vi "PH_Trendviewer_Powermeter.ProcCases.vi"(0 "i ref in":refnum<vi>, 1 "selector":string, 2 "Data":T1, 3 "call cluster":T2={"Object"="", "Selector"="", "CallType"=enum."synchronous", "Async Object"="", "Async Selector"="", "Data Descriptor"="", "Data"=[], "Error #"=0, "Expire"=0}, 5 "error in (no error)":errorcluster) -> (14 "i ref out":refnum<vi>, 17 "answer cluster":T2={"Object"="", "Selector"="", "CallType"=enum."synchronous", "Async Object"="", "Async Selector"="", "Data Descriptor"="", "Data"=[], "Error #"=0, "Expire"=0}, 19 "error out":errorcluster)   [LabVIEW 2014, in "PH_Trendviewer_Powermeter.lvlib"]
doc: "This method is called by a process from within the default case in the event loop. The methods of a class that are linked to events will be called from THIS method. Add your code here."
uses:
  PH_Trendviewer_Powermeter.lvlib
  CS_Core/CSSystem/CoreDefs/CoreDefs.call_type.ctl
  CS_Core/BaseProcess/BaseProcess.descriptor string definition.ctl
  CS_Core/CSSystem/CoreDefs/CoreDefs.rawDataType.ctl
  CS_Core/CSSystem/CoreLib/CoreLib.byte array 2 short.vi
  CS_Core/CSSystem/CoreLib/CoreLib.string 2 byte array.vi
  CS_Core/CSSystem/CoreLib/CoreLib.lvlib
  CS_Core/BaseProcess/BaseProcess.lvlib
  PH_Basics/PH_PSDBWriter/PH_PSDBWriter.lvlib
  CS_Core/CAEObj/CAEObj.lvlib
  PH_Basics/PH_Common/PH_Common.lvlib
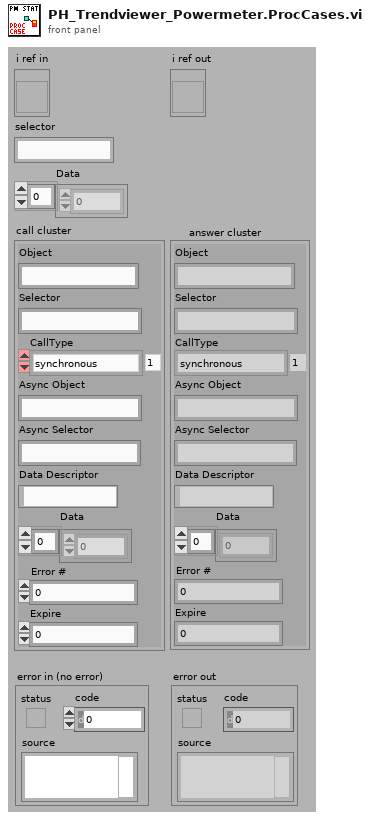
[diagram p1: front panel]
types:
  T1 = typedef "CoreDefs.rawDataType.ctl" = i8[]
  T2 = typedef "CoreDefs.call_type.ctl" = cluster{"Object":string, "Selector":string, "CallType":enum16{"simple", "synchronous", "asynchronous"}, "Async Object":string, "Async Selector":string, "Data Descriptor":T3, "Data":T1, "Error #":i32, "Expire":u32}
  T3 = typedef "BaseProcess.lvlib/BaseProcess.descriptor string definition.ctl" = string
  T4 = typedef "PH_Trendviewer_Powermeter.lvlib/PH_Trendviewer_Powermeter.i attribute.ctl" = cluster{"GUI Refs ":cluster{"Status":refnum<vi>, "Result Graph":refnum<vi>, "Mean Data":refnum<vi>, "Std Dev Data":refnum<vi>, "Dummy Mean":refnum<vi>, "Dummy Std Dev":refnum<vi>, "Export Data":refnum<vi>, "Stat or Trend":refnum<vi>, "Delete":refnum<vi>, "Powermeter":refnum<vi>, "Start":refnum<vi>}, "Powermeter":string, "Stat or Trend":bool, "Start":bool, "Data":cluster{"Time Stamp":timestamp, "Energy [J]":dbl}[], "Datasets strored":i32, "Dataarray Size":i32}
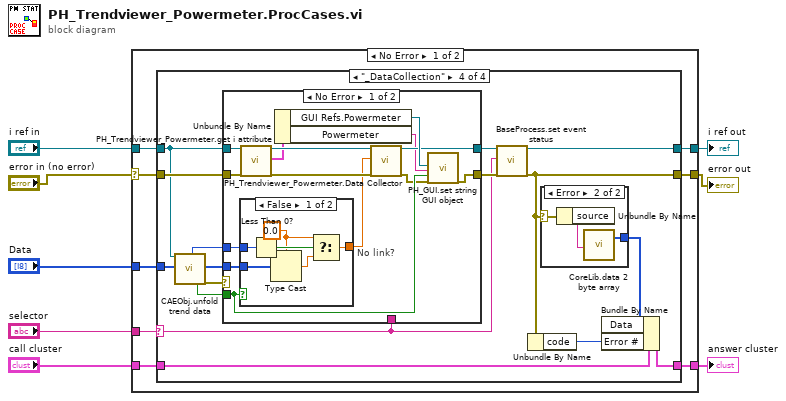
[diagram p0: block diagram]
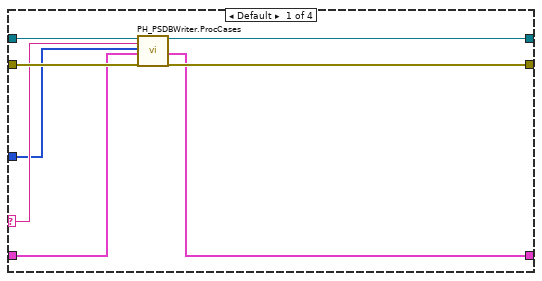
[diagram p2: hidden frame]
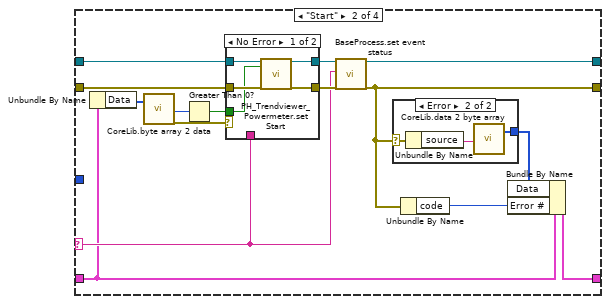
[diagram p3: hidden frame]
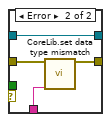
[diagram p5: hidden frame]
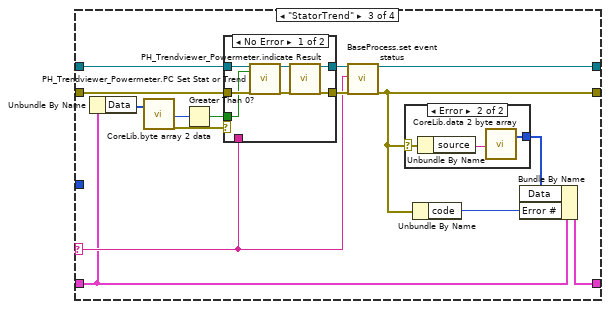
[diagram p6: hidden frame]
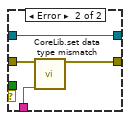
[diagram p8: hidden frame]
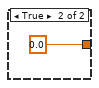
[diagram p10: hidden frame]
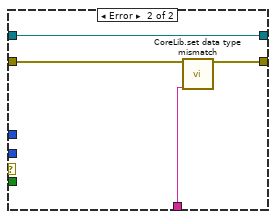
[diagram p11: hidden frame]
diagram:
  n1 = case shown="No Error" "error in (no error)" {
    selector: "error in (no error)" -> [w9 w126]
    tunnel: "selector" -> [w16 _]
    tunnel: [w15 w125] -> w7
    tunnel: "call cluster" -> [w14 w125]
    tunnel: "i ref in" -> [w13 w127]
    tunnel: [w12 w127] -> w5
    tunnel: [w11 w126] -> w4
    tunnel: "Data" -> [w10 _]
    frame No Error {
      n2 = case shown="\"_DataCollection\"" w16 {
        selector: w16 -> [w19 w28 w55 w89]
        tunnel: w13 -> [w18 w32 w59 w85]
        tunnel: [w24 w30 w57 w91] -> w12
        tunnel: w14 -> [w20 w27 w54 w88]
        tunnel: [w21 w26 w53 w87] -> w15
        tunnel: w9 -> [w23 w31 w58 w92]
        tunnel: [w22 w29 w56 w90] -> w11
        tunnel: w10 -> [w17 _ _ w86]
        frame Default {
          n3 = call "PH_PSDBWriter.ProcCases.vi"("i ref in"=w18, "selector"=w19, "Data"=w17, "call cluster"=w20, "error in"=w23) -> ("i ref out"=w24:refnum<vi>, "answer cluster"=w21:T2, "error out"=w22:errorcluster)  [unwired: 12 in]
        }
        frame "Start" {
          n4 = Unbundle By Name(w27) -> ("Data"=w35:T1)
          n5 = call-poly "CoreLib.byte array 2 data.vi"("byteArray"=w35) -> ("i16"=w36:i16, "error out"=w25:errorcluster)  [unwired: 16 in, 1 out]
          n6 = Greater Than 0?(x=w36) -> (x > 0?=w37:bool)
          n7 = case shown="No Error" w25 {
            tunnel: [w47 w51] -> w33
            tunnel: w32 -> [w46 w51]
            tunnel: w31 -> [w45 w50]
            tunnel: [w44 w49] -> w34
            tunnel: w28 -> [_ w48]
            tunnel: w37 -> [w43 _]
            frame No Error {
              n8 = call "PH_Trendviewer_Powermeter.set Start.vi"("i ref in"=w46, "Start"=w43, "error in (no error)"=w45) -> ("i ref out"=w47:refnum<vi>, "error out"=w44:errorcluster)  [unwired: 15 in]
            }
            frame Error {
              n9 = call "CoreLib.set data type mismatch.vi"("error in (no error)"=w50, "error source"=w48) -> ("error out"=w49:errorcluster)  [unwired: 17 in]
            }
          }
          n10 = call "BaseProcess.set event status.vi"("i ref in"=w33, "EventStatus"=w28, "error in (no error)"=w34) -> ("i ref out"=w30:refnum<vi>, "error out"=w29:errorcluster)  [unwired: 14 in, 1 out]
          n11 = case shown="Error" w29 {
            selector: w29 -> [_ w42]
            tunnel: [_ w40] -> w39
            frame No Error {
            }
            frame Error {
              n12 = Unbundle By Name(w42) -> ("source"=w41:string)
              n13 = call-poly "CoreLib.data 2 byte array.vi"("string"=w41) -> ("byteArray out"=w40:T1)  [unwired: 18 in]
            }
          }
          n14 = Unbundle By Name(w29) -> ("code"=w38:i32)
          n15 = Bundle By Name(cluster=w27, "Data"=w39, "Error #"=w38) -> (w26:T2)
        }
        frame "StatorTrend" {
          n16 = Unbundle By Name(w54) -> ("Data"=w62:T1)
          n17 = call-poly "CoreLib.byte array 2 data.vi"("byteArray"=w62) -> ("i16"=w63:i16, "error out"=w52:errorcluster)  [unwired: 16 in, 1 out]
          n18 = Greater Than 0?(x=w63) -> (x > 0?=w64:bool)
          n19 = case shown="No Error" w52 {
            tunnel: [w72 w80] -> w60
            tunnel: w59 -> [w76 w80]
            tunnel: w58 -> [w75 w79]
            tunnel: [w70 w78] -> w61
            tunnel: w55 -> [_ w77]
            tunnel: w64 -> [w74 _]
            frame No Error {
              n20 = call "PH_Trendviewer_Powermeter.PC Set Stat or Trend.vi"("i ref in"=w76, "Stat or Trend"=w74, "error in (no error)"=w75) -> ("i ref out"=w73:refnum<vi>, "error out"=w71:errorcluster)  [unwired: 15 in]
              n21 = call "PH_Trendviewer_Powermeter.indicate Result.vi"("i ref in"=w73, "error in (no error)"=w71) -> ("i ref out"=w72:refnum<vi>, "error out"=w70:errorcluster)  [unwired: 16 in]
            }
            frame Error {
              n22 = call "CoreLib.set data type mismatch.vi"("error in (no error)"=w79, "error source"=w77) -> ("error out"=w78:errorcluster)  [unwired: 17 in]
            }
          }
          n23 = call "BaseProcess.set event status.vi"("i ref in"=w60, "EventStatus"=w55, "error in (no error)"=w61) -> ("i ref out"=w57:refnum<vi>, "error out"=w56:errorcluster)  [unwired: 14 in, 1 out]
          n24 = case shown="Error" w56 {
            selector: w56 -> [_ w69]
            tunnel: [_ w67] -> w66
            frame No Error {
            }
            frame Error {
              n25 = Unbundle By Name(w69) -> ("source"=w68:string)
              n26 = call-poly "CoreLib.data 2 byte array.vi"("string"=w68) -> ("byteArray out"=w67:T1)  [unwired: 18 in]
            }
          }
          n27 = Unbundle By Name(w56) -> ("code"=w65:i32)
          n28 = Bundle By Name(cluster=w54, "Data"=w66, "Error #"=w65) -> (w53:T2)
        }
        frame "_DataCollection" {
          n29 = call "CAEObj.unfold trend data.vi"("i ref in"=w85, "raw trend data"=w86) -> ("quality"=w81:i32, "no link"=w83:bool, "data"=w82:i8[], "error out"=w84:errorcluster)  [unwired: 9 in, 5 out]
          n30 = case shown="No Error" w84 {
            tunnel: [w108 w124] -> w93
            tunnel: w85 -> [w105 w124]
            tunnel: w92 -> [w106 w123]
            tunnel: [w111 w122] -> w94
            tunnel: w89 -> [_ w121]
            tunnel: w83 -> [w110 _]
            tunnel: w82 -> [w113 _]
            tunnel: w81 -> [w112 _]
            frame No Error {
              n31 = case "No link?" shown="False" w110 {
                tunnel: [w115 0.0] -> w101
                tunnel: w112 -> [w119 _]
                tunnel: w113 -> [w118 _]
                frame False {
                  w114 = 0.0
                  n32 = Less Than 0?(x=w119) -> (x < 0?=w117:bool)
                  n33 = Type Cast(type=w114, x=w118) -> (*(type *) &x=w116:dbl)
                  n34 = Select(t=w114, s=w117, f=w116) -> (s? t:f=w115:dbl)
                }
                frame True {
                }
              }
              n35 = call "PH_Trendviewer_Powermeter.get i attribute.vi"("i ref in"=w105, "error in (no error)"=w106) -> ("i ref out"=w104:refnum<vi>, "i attribute"=w102:T4, "error out"=w103:errorcluster)  [unwired: 15 in]
              n36 = Unbundle By Name(w102) -> ("GUI Refs.Powermeter"=w109:refnum<vi>, "Powermeter"=w100:string)
              n37 = call "PH_Trendviewer_Powermeter.Data Collector.vi"("i ref in"=w104, "Energy [J]"=w101, "error in (no error)"=w103) -> ("i ref out"=w108:refnum<vi>, "error out"=w107:errorcluster)  [unwired: 15 in]
              n38 = call "PH_GUI.set string GUI object.vi"("GUI object Ref"=w109, "Text"=w100, "Blinking? (false)"=w110, "error in"=w107) -> ("error out"=w111:errorcluster)  [unwired: 15 in]
            }
            frame Error {
              n39 = call "CoreLib.set data type mismatch.vi"("error in (no error)"=w123, "error source"=w121) -> ("error out"=w122:errorcluster)  [unwired: 17 in]
            }
          }
          n40 = call "BaseProcess.set event status.vi"("i ref in"=w93, "EventStatus"=w89, "error in (no error)"=w94) -> ("i ref out"=w91:refnum<vi>, "error out"=w90:errorcluster)  [unwired: 14 in, 1 out]
          n41 = Unbundle By Name(w90) -> ("code"=w95:i32)
          n42 = case shown="Error" w90 {
            selector: w90 -> [_ w99]
            tunnel: [_ w97] -> w96
            frame No Error {
            }
            frame Error {
              n43 = Unbundle By Name(w99) -> ("source"=w98:string)
              n44 = call-poly "CoreLib.data 2 byte array.vi"("string"=w98) -> ("byteArray out"=w97:T1)  [unwired: 18 in]
            }
          }
          n45 = Bundle By Name(cluster=w88, "Data"=w96, "Error #"=w95) -> (w87:T2)
        }
      }
    }
    frame Error {
    }
  }
  "answer cluster" <- w7
  "i ref out" <- w5
  "error out" <- w4
